vi "Split cluster or array pyhton string.vi"(8 "error in (no error)":errorcluster, 9 "offset":i32, 10 "Comma Delimited Python Data":string) -> (0 "error out":errorcluster, 1 "offset past element":i32, 2 "Remaining Elements":string, 3 "First Element":string, 4 "Has Remaining Elements":bool)   [LabVIEW 2020, in "jki_python_data_tools.lvlib"]
uses:
  jki_python_data_tools.lvlib
  <vilib>/regexp/Match Regular Expression.xnode
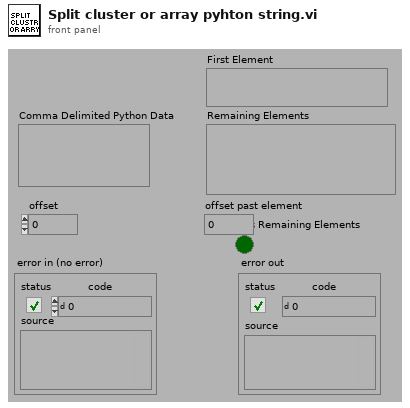
[diagram p1: front panel]
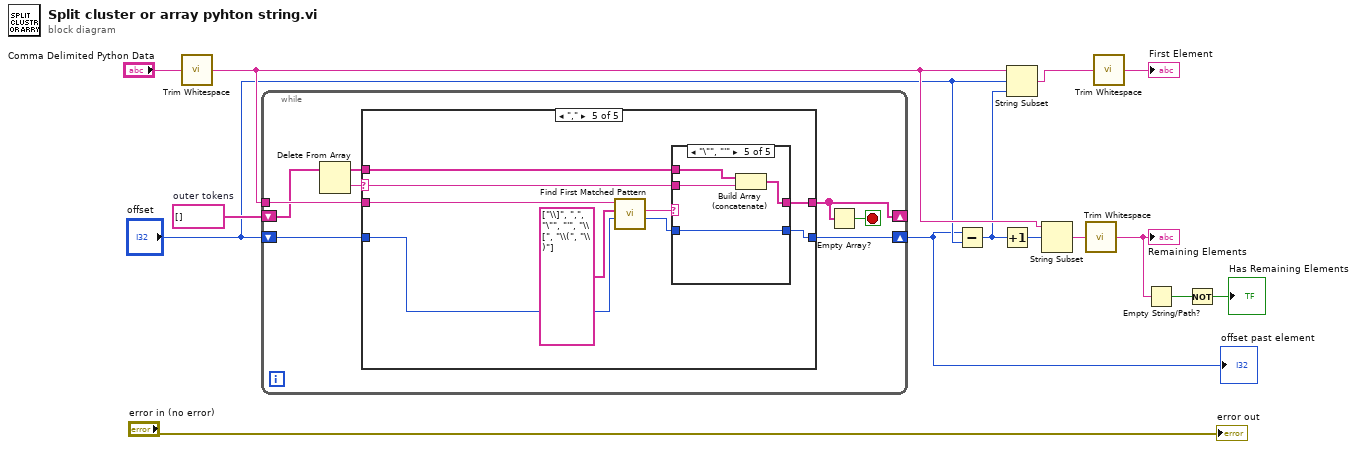
[diagram p0: block diagram]
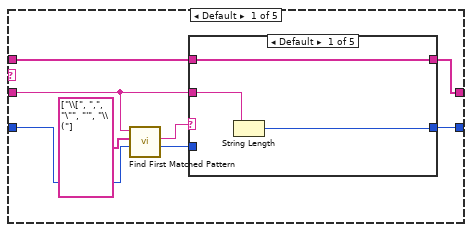
[diagram p2: hidden frame]
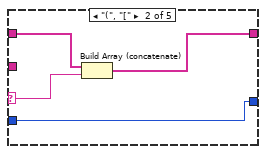
[diagram p3: hidden frame]
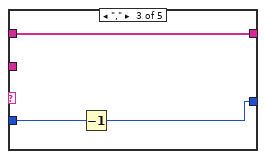
[diagram p4: hidden frame]
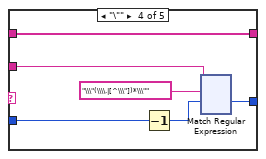
[diagram p5: hidden frame]
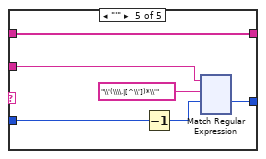
[diagram p6: hidden frame]
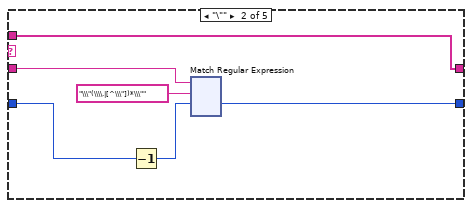
[diagram p7: hidden frame]
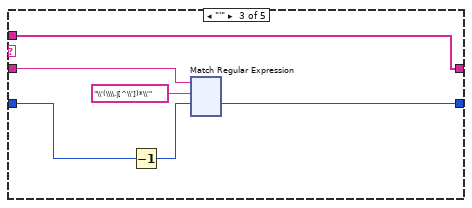
[diagram p8: hidden frame]
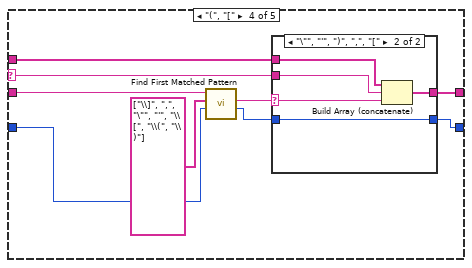
[diagram p9: hidden frame]
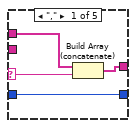
[diagram p11: hidden frame]
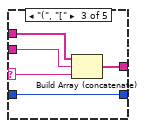
[diagram p13: hidden frame]
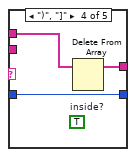
[diagram p14: hidden frame]
diagram:
  w5 = string[] []  # outer tokens
  n1 = call <vilib>:"Trim Whitespace.vi"("string"="Comma Delimited Python Data") -> ("trimmed string"=w9:string)  [unwired: 1 in]
  n2 = while {
    tunnel: w9 -> [w22]
    shift-right: [w18] -> _
    shift-left: w5 -> [w21]
    shift-right: [w19] -> w2
    shift-left: "offset" -> [w20]
    stop <- w17 stop-if-true
    n3 = Delete From Array(array=w21) -> (deleted portion=w16:string, array with subset deleted=w15:string[])  [unwired: 2 in]
    n4 = case shown="\",\"" w16 {
      selector: w16 -> [_ _ _ w528 w542]
      tunnel: w20 -> [w23 w284 w404 w522 w538]
      tunnel: w22 -> [w27 w285 w405 w525 w545]
      tunnel: [w29 w283 w403 w527 w541] -> w19
      tunnel: w15 -> [w30 w282 w402 w529 w544]
      tunnel: [w28 w282 w402 w526 w540] -> w18
      frame Default {
        n5 = call "Find First Matched Pattern.vi"("Numeric in"=w23, "RE characters to match (must be pre-escaped)"=string[] ["\\[", ",", "\"", "'", "\\("], "trimmed string in"=w27) -> ("offset past match"=w24:i32, "match"=w26:string)  [unwired: 7 in]
        n6 = case shown="Default" w26 {
          selector: w26 -> [_ w36 _ _ _]
          tunnel: [w31 w34 w38 w44 w164] -> w29
          tunnel: w30 -> [w33 w37 w40 w46 w166]
          tunnel: [w33 w35 w40 w46 w166] -> w28
          tunnel: w24 -> [_ w34 w39 w43 w163]
          tunnel: w27 -> [w32 _ _ w41 w161]
          frame Default {
            n7 = String Length(string=w32) -> (length=w31:i32)
          }
          frame "(", "[" {
            n8 = Build Array (concatenate)(w37, w36) -> (w35:string[])
          }
          frame "," {
            n9 = Decrement(x=w39) -> (x-1=w38:i32)
          }
          frame "\"" {
            n10 = Decrement(x=w43) -> (x-1=w42:i32)
            n11 = xnode "Match Regular Expression"("input string"=w41, "regular expression"="\\\"(\\\\.|[^\\\"])*\\\"", "offset (0)"=w42) -> ("offset past match"=w44:i32)  [unwired: 3 in, 4 out]
          }
          frame "'" {
            n12 = Decrement(x=w163) -> (x-1=w162:i32)
            n13 = xnode "Match Regular Expression"("input string"=w161, "regular expression"="\\'(\\\\.|[^\\'])*\\'", "offset (0)"=w162) -> ("offset past match"=w164:i32)  [unwired: 3 in, 4 out]
          }
        }
      }
      frame "\"" {
        n14 = Decrement(x=w284) -> (x-1=w281:i32)
        n15 = xnode "Match Regular Expression"("input string"=w285, "regular expression"="\\\"(\\\\.|[^\\\"])*\\\"", "offset (0)"=w281) -> ("offset past match"=w283:i32)  [unwired: 3 in, 4 out]
      }
      frame "'" {
        n16 = Decrement(x=w404) -> (x-1=w401:i32)
        n17 = xnode "Match Regular Expression"("input string"=w405, "regular expression"="\\'(\\\\.|[^\\'])*\\'", "offset (0)"=w401) -> ("offset past match"=w403:i32)  [unwired: 3 in, 4 out]
      }
      frame "(", "[" {
        n18 = call "Find First Matched Pattern.vi"("Numeric in"=w522, "RE characters to match (must be pre-escaped)"=string[] ["\\]", ",", "\"", "'", "\\[", "\\(", "\\)"], "trimmed string in"=w525) -> ("offset past match"=w521:i32, "match"=w524:string)  [unwired: 7 in]
        n19 = case shown="\"\\\"\", \"'\", \")\", \",\", \"[\"" w524 {
          selector: w524 -> [_ w532]
          tunnel: w529 -> [w531 w536]
          tunnel: w528 -> [_ w535]
          tunnel: [w530 w534] -> w527
          tunnel: w521 -> [w530 w534]
          tunnel: [w531 w533] -> w526
          frame Default {
          }
          frame "\"", "'", ")", ",", "[" {
            n20 = Build Array (concatenate)(w536, w535, w532) -> (w533:string[])
          }
        }
      }
      frame "," {
        n21 = call "Find First Matched Pattern.vi"("Numeric in"=w538, "RE characters to match (must be pre-escaped)"=string[] ["\\]", ",", "\"", "'", "\\[", "\\(", "\\)"], "trimmed string in"=w545) -> ("offset past match"=w539:i32, "match"=w543:string)  [unwired: 7 in]
        n22 = case shown="\"\\\"\", \"'\"" w543 {
          selector: w543 -> [w547 _ w550 _ _]
          tunnel: w544 -> [w549 _ w554 w556 w561]
          tunnel: w542 -> [_ _ w553 _ w560]
          tunnel: [w546 _ w552 w557 w559] -> w541
          tunnel: w539 -> [w546 _ w552 w557 w559]
          tunnel: [w548 _ w551 w555 w558] -> w540
          frame "," {
            n23 = Build Array (concatenate)(w549, w547) -> (w548:string[])
          }
          frame Default {
          }
          frame "(", "[" {
            n24 = Build Array (concatenate)(w554, w553, w550) -> (w551:string[])
          }
          frame ")", "]" {
            (unwired) TRUE  # inside?
            n25 = Delete From Array(array=w556) -> (array with subset deleted=w555:string[])  [unwired: 2 in, 1 out]
          }
          frame "\"", "'" {
            n26 = Build Array (concatenate)(w561, w560) -> (w558:string[])
          }
        }
      }
    }
    n27 = Empty Array?(array=w18) -> (empty?=w17:bool)
  }
  "offset past element" <- w2
  n28 = Subtract(x=w2, y="offset") -> (x-y=w1:i32)
  n29 = Increment(x=w1) -> (x+1=w4:i32)
  n30 = String Subset(string=w9, offset (0)="offset", length (rest)=w1) -> (substring=w8:string)
  n31 = String Subset(string=w9, offset (0)=w4) -> (substring=w6:string)  [unwired: 1 in]
  n32 = call <vilib>:"Trim Whitespace.vi"("string"=w6) -> ("trimmed string"=w13:string)  [unwired: 1 in]
  "Remaining Elements" <- w13
  n33 = call <vilib>:"Trim Whitespace.vi"("string"=w8) -> ("trimmed string"=→"First Element":string)  [unwired: 1 in]
  n34 = Empty String/Path?(string/path=w13) -> (empty?=w12:bool)
  n35 = Not(x=w12) -> (.not. x?=→"Has Remaining Elements":bool)
  "error out" <- "error in (no error)"
